vi "Write Excel Files.vi"() -> ()   [LabVIEW 2016]
uses:
  <vilib>/Utility/NIReport.llb/NI_report.lvclass
  sdi_12/Groundwater header.ctl
  <userlib>/_OpenG.lib/file/file.llb/File Exists - Scalar__ogtk.vi
  <userlib>/_OpenG.lib/file/file.llb/Strip Path - Traditional__ogtk.vi
  <vilib>/Utility/file.llb/Write Delimited Spreadsheet (string).vi
  <vilib>/Utility/file.llb/Read Delimited Spreadsheet (string).vi
panel:
  in  "Output path to Directory":path=path "C:/Cascade/Data/Output Files/ara-1"
  in  "Sonde Calibration History File":path
  out "IK Reason array":string[][](array[string])
  in  "Sonde IK Recording Failure Path":path
  out "Recording Reason Sonde array":string[][](array[string])
  in  "Temporary Data Files Directory":path=path "C:/Cascade/Data/Output Files"
  out "KPRO all rows":string[][](array[string])
  out "Sonde Data":string[][](array[string])
  out "Sonde Recording":string[][](array[string])
  out "IK":string[][](array[string])
  out "appended path":path=path "C:/Cascade/Data/Output Files/ara-1/ara-1"
  out "Down hole Pressure Transducer CSV data  path":path=path "C:/Cascade/Data/Output Files/ara-1/ara-1_DHT Data.csv"
  in  "Static IK path":path=path "C:/Cascade/Data/Output Files/ara-1/ara-1_Static Ik.csv"
  out "Output File Path":path=path "C:/Cascade/Data/Output Files/ara-1"
  out "KPRO SessionOutput File Path":path=path "C:/Cascade/Data/Output Files/ara-1/ara-1_KPROsession.csv"
  in  "Sonde Recording Error file":path=path "C:/Cascade/Data/Output Files/ara-1/ara-1_Sample failure.csv"
  in  "IK Recording Error file":path=path "C:/Cascade/Data/Output Files/ara-1/ara-1_IK failure.csv"
  in  "Sonde Output File Path":path=path "C:/Cascade/Data/Output Files/ara-1/ara-1_SondeData.csv"
  in  "KPRO Cumulative Output File Path":path=path "C:/Cascade/Data/Output Files/ara-1/ara-1_KPROcumulative.csv"
  out "error out":errorcluster
  in  "error IO":errorcluster
  in  "Groundwater Header":T1
  in  "Excel report file path":path=path "C:/Cascade/Data/Excel Reports/Groundwater Profiling Log_ara1.xlsx"
  in  "template file path":path=path "C:/Cascade/templates/Groundwater Profiling Log_empty_labview_template.xlsx"
  out "Worksheet Names":string[](array[string])
  out "row max value":i32
  in  "Header path":path=path "C:/Cascade/templates/Fields for Excel sheets.xlsx"
  out "column max value":i32
  out "subarray":string[][](array[string])
  out "NI_report out":refnum<class "NI_report.lvclass">
  out "Number of Sample Sheets":i32
  out "Select Worksheet Index":i32
  out "Columns":i32[](array[numeric])
  out "Column of Volume":i32
  out "last occupied cell's name":string
  in  "Current Sample Sheet":string="Sample 1"
types:
  T1 = typedef "Groundwater header.ctl" = cluster{"Location":string, "Date Finished":string, "CTS":string, "sampler":string, "Kpro box Serial ":string, "Sonde Serial":string, "Drilling Contractor":string, "Ave Depth to Water":string, "Gas/Peri Pump":string, "Atmospheric Pressure":string, "KPRO N2 Pressure":string, "Gas Drive N2 Pressure":string, "Profile ID":string, "Client":string}
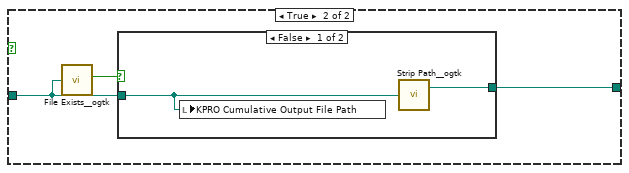
[diagram p2: hidden frame]
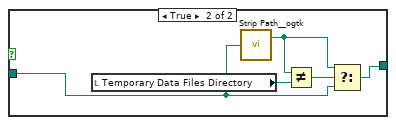
[diagram p3: hidden frame]
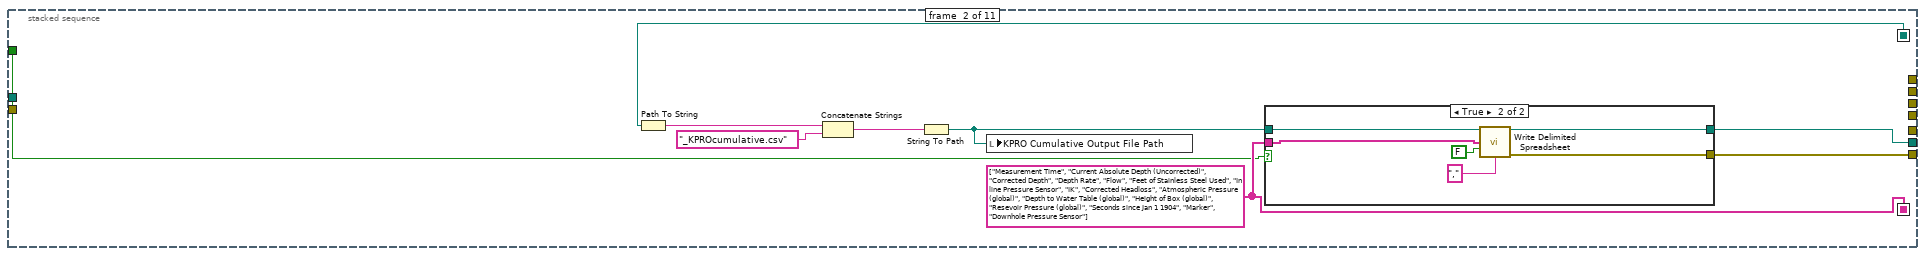
[diagram p4: hidden frame]
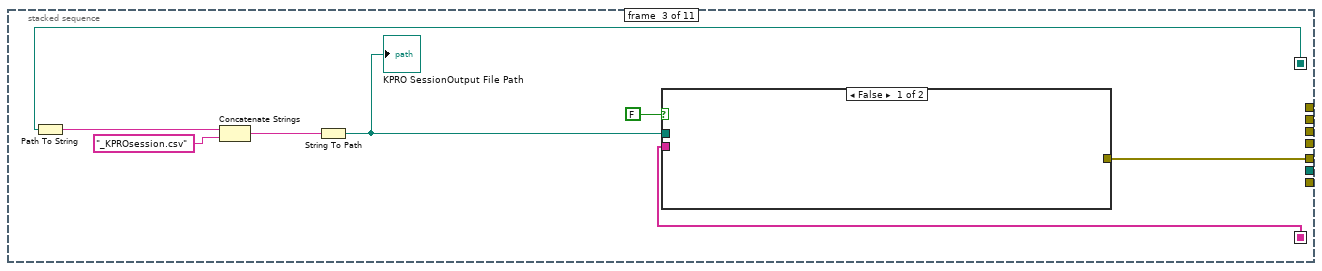
[diagram p6: hidden frame]
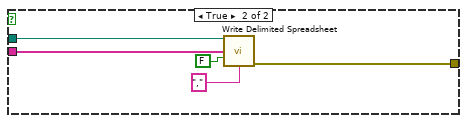
[diagram p7: hidden frame]
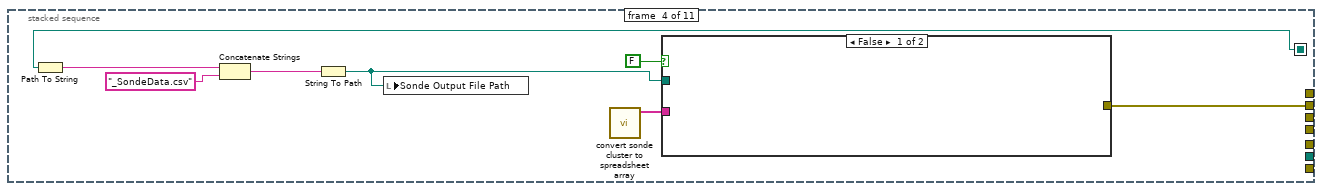
[diagram p8: hidden frame]
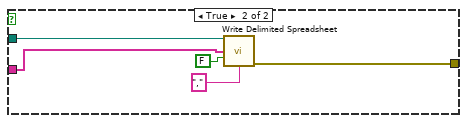
[diagram p9: hidden frame]
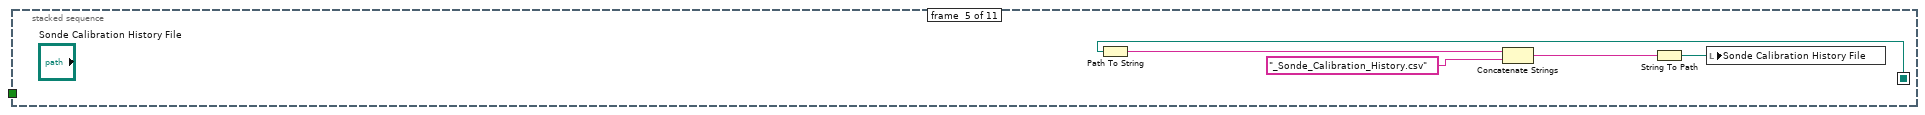
[diagram p10: hidden frame]
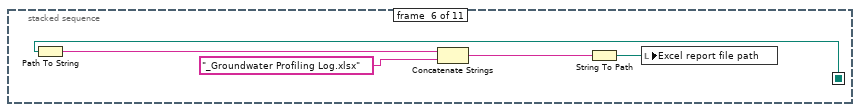
[diagram p11: hidden frame]
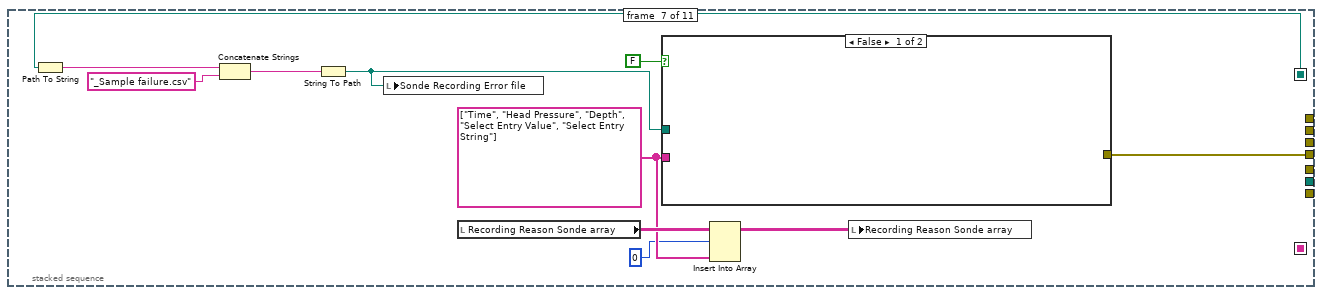
[diagram p12: hidden frame]
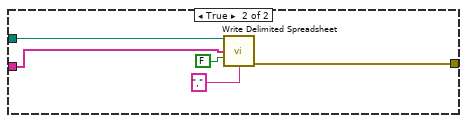
[diagram p13: hidden frame]
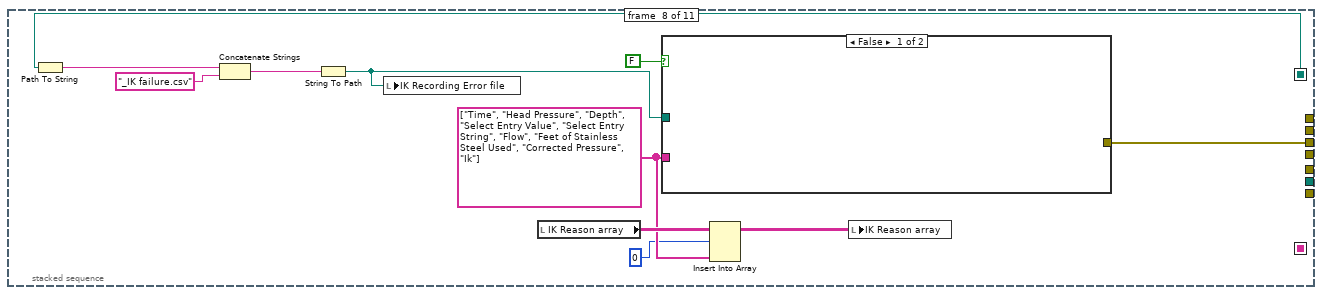
[diagram p14: hidden frame]
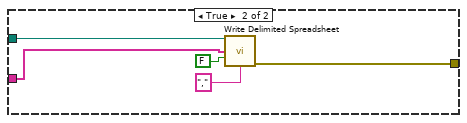
[diagram p15: hidden frame]
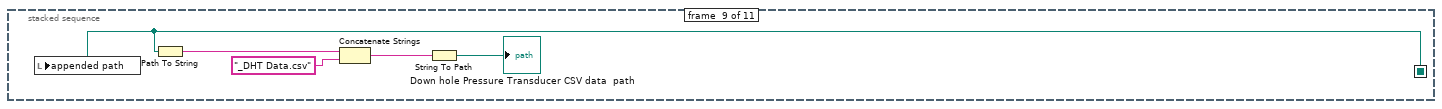
[diagram p16: hidden frame]
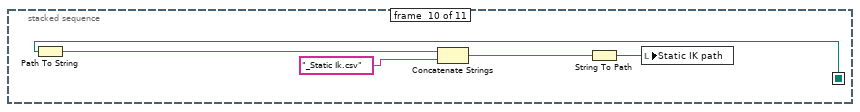
[diagram p17: hidden frame]
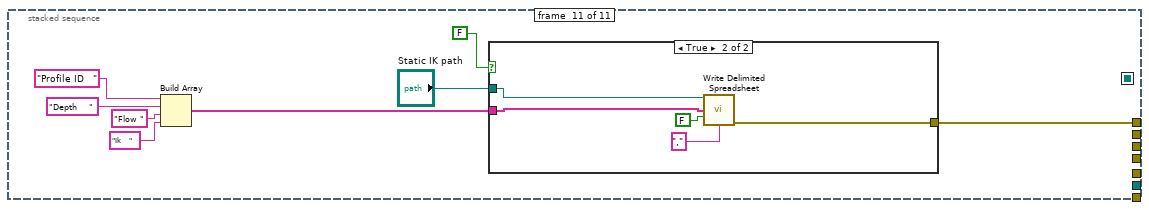
[diagram p18: hidden frame]
diagram:
  w14 = "Groundwater Profile Log" ("Worksheet Name in")
  w31 = "Profile Info" ("Worksheet Name in")
  n1 = stacked-sequence {
    seq-local: [_ w86 _ _ _ _ _ _ _ _ _] -> [_ _ w101 _ _ _ _ _ _ _ _]
    seq-local: [w62 _ _ _ _ _ _ _ _ _ _] -> [_ w87 w102 w114 w125 w130 w141 w157 w168 w172 _]
    tunnel: [_ w84 _ _ _ _ _ _ _ _ _] -> w1
    tunnel: [_ _ w106 _ _ _ _ _ _ _ _] -> _
    tunnel: [_ _ _ w115 _ _ _ _ _ _ _] -> _
    tunnel: [_ _ _ _ _ _ w142 _ _ _ _] -> _
    tunnel: [_ _ _ _ _ _ _ w158 _ _ _] -> _
    tunnel: [_ _ _ _ _ _ _ _ _ _ w179] -> _
    tunnel: [_ w88 _ _ _ _ _ _ _ _ _] -> _
    tunnel: "Output path to Directory" -> [w65 _ _ _ _ _ _ _ _ _ _]
    tunnel: FALSE ("exists") -> [w66 w85 _ _ _ _ _ _ _ _ _]
    tunnel: "error IO" -> [_ _ _ _ _ _ _ _ _ _ _]
    frame #0 {
      n2 = case shown="False" w66 {
        tunnel: w65 -> [w72 w74]
        tunnel: [w72 w73] -> w64
        frame False {
        }
        frame True {
          n3 = call-poly <userlib>:"File Exists__ogtk.vi"("file path"=w74) -> ("is directory"=w75:bool)  [unwired: 6 in, 1 out]
          n4 = case shown="False" w75 {
            tunnel: w74 -> [w76 w78]
            tunnel: [w77 w79] -> w73
            frame False {
              n5 = local write "KPRO Cumulative Output File Path"(w76) -> ()
              n6 = call-poly <userlib>:"Strip Path__ogtk.vi"("path"=w76) -> ("stripped path"=w77:path)  [unwired: 1 out]
            }
            frame True {
              n7 = local read "Temporary Data Files Directory"() -> (w82:path)
              n8 = call-poly <userlib>:"Strip Path__ogtk.vi"("path"=w78) -> ("stripped path"=w80:path)  [unwired: 1 out]
              n9 = Not Equal?(x=w80, y=w82) -> (x != y?=w81:bool)
              n10 = Select(t=w80, s=w81, f=w78) -> (s? t:f=w79:path)
            }
          }
        }
      }
      n11 = Path To String(path=w64) -> (string=w69:string)
      n12 = Concatenate Strings(w69, "\\" ("string")) -> (w70:string)
      n13 = String To Path(string=w70) -> (path=w63:path)
      "Output File Path" <- w63
      n14 = call-poly <userlib>:"Strip Path__ogtk.vi"("path"=w63) -> ("name"=w67:string)  [unwired: 1 out]
      n15 = Concatenate Strings(w70, w67) -> (w68:string)
      n16 = String To Path(string=w68) -> (path=w62:path)
      "appended path" <- w62
    }
    frame #1 {
      w86 = string[] ["Measurement Time", "Current Absolute Depth (Uncorrected)", "Corrected Depth", "Depth Rate", "Flow", "Feet of Stainless Steel Used", "In line Pressure Sensor", "IK", "Corrected Headloss", "Atmospheric Pressure (global)", "Depth to Water Table (global)", "Height of Box (global)", "Resevoir Pressure (global)", "Seconds since Jan 1 1904", "Marker", "Downhole Pressure Sensor"] ("Array")
      n17 = Path To String(path=w87) -> (string=w89:string)
      n18 = Concatenate Strings(w89, "_KPROcumulative.csv") -> (w91:string)
      n19 = String To Path(string=w91) -> (path=w83:path)
      n20 = local write "KPRO Cumulative Output File Path"(w83) -> ()
      n21 = case shown="True" w85 {
        tunnel: [_ w96] -> w84
        tunnel: w83 -> [w92 w95]
        tunnel: [w92 w94] -> w88
        tunnel: w86 -> [_ w93]
        frame False {
        }
        frame True {
          n22 = call-poly <vilib>:"Write Delimited Spreadsheet.vi"("file path (dialog if empty)"=w95, "1D data"=w93, "append to file? (new file:F)"=FALSE, "delimiter (\\t)"="," ("delimiter (\\t)")) -> ("new file path (Not A Path if cancelled)"=w94:path, "error out"=w96:errorcluster)  [unwired: 10 in]
        }
      }
    }
    frame #2 {
      n23 = Path To String(path=w102) -> (string=w104:string)
      n24 = Concatenate Strings(w104, "_KPROsession.csv") -> (w105:string)
      n25 = String To Path(string=w105) -> (path=w100:path)
      "KPRO SessionOutput File Path" <- w100
      n26 = case shown="False" FALSE {
        tunnel: [_ w109] -> w106
        tunnel: w101 -> [_ w108]
        tunnel: w100 -> [_ w107]
        frame False {
        }
        frame True {
          n27 = call-poly <vilib>:"Write Delimited Spreadsheet.vi"("file path (dialog if empty)"=w107, "1D data"=w108, "append to file? (new file:F)"=FALSE, "delimiter (\\t)"="," ("delimiter (\\t)")) -> ("error out"=w109:errorcluster)  [unwired: 10 in, 1 out]
        }
      }
    }
    frame #3 {
      n28 = Path To String(path=w114) -> (string=w117:string)
      n29 = Concatenate Strings(w117, "_SondeData.csv" ("string")) -> (w118:string)
      n30 = String To Path(string=w118) -> (path=w113:path)
      n31 = local write "Sonde Output File Path"(w113) -> ()
      n32 = call "convert sonde cluster to spreadsheet array.vi"() -> ("sonde labels"=w116:string[])  [unwired: 8 in, 3 out]
      n33 = case shown="False" FALSE {
        tunnel: w116 -> [_ w124]
        tunnel: [_ w121] -> w115
        tunnel: w113 -> [_ w120]
        frame False {
        }
        frame True {
          n34 = call-poly <vilib>:"Write Delimited Spreadsheet.vi"("file path (dialog if empty)"=w120, "1D data"=w124, "append to file? (new file:F)"=FALSE, "delimiter (\\t)"="," ("delimiter (\\t)")) -> ("error out"=w121:errorcluster)  [unwired: 10 in, 1 out]
        }
      }
    }
    frame #4 {
      n35 = Path To String(path=w125) -> (string=w127:string)
      n36 = Concatenate Strings(w127, "_Sonde_Calibration_History.csv" ("string")) -> (w128:string)
      n37 = String To Path(string=w128) -> (path=w126:path)
      n38 = local write "Sonde Calibration History File"(w126) -> ()
    }
    frame #5 {
      n39 = Path To String(path=w130) -> (string=w132:string)
      n40 = Concatenate Strings(w132, "_Groundwater Profiling Log.xlsx" ("string")) -> (w133:string)
      n41 = String To Path(string=w133) -> (path=w131:path)
      n42 = local write "Excel report file path"(w131) -> ()
    }
    frame #6 {
      w138 = string[] ["Time", "Head Pressure", "Depth", "Select Entry Value", "Select Entry String"]
      n43 = Path To String(path=w141) -> (string=w143:string)
      n44 = Concatenate Strings(w143, "_Sample failure.csv" ("new ending (none)")) -> (w144:string)
      n45 = String To Path(string=w144) -> (path=w136:path)
      n46 = local write "Sonde Recording Error file"(w136) -> ()
      n47 = local read "Recording Reason Sonde array"() -> (w139:string[][])
      n48 = case shown="False" FALSE {
        tunnel: [_ w148] -> w142
        tunnel: w138 -> [_ w147]
        tunnel: w136 -> [_ w146]
        frame False {
        }
        frame True {
          n49 = call-poly <vilib>:"Write Delimited Spreadsheet.vi"("file path (dialog if empty)"=w146, "1D data"=w147, "append to file? (new file:F)"=FALSE, "delimiter (\\t)"="," ("delimiter (\\t)")) -> ("error out"=w148:errorcluster)  [unwired: 10 in, 1 out]
        }
      }
      n50 = Insert Into Array(array=w139, index (row)=0, new element=w138) -> (w140:string[][])  [unwired: 1 in]
      n51 = local write "Recording Reason Sonde array"(w140) -> ()
    }
    frame #7 {
      w154 = string[] ["Time", "Head Pressure", "Depth", "Select Entry Value", "Select Entry String", "Flow", "Feet of Stainless Steel Used", "Corrected Pressure", "Ik"]
      n52 = Path To String(path=w157) -> (string=w159:string)
      n53 = Concatenate Strings(w159, "_IK failure.csv" ("new ending (none)")) -> (w160:string)
      n54 = String To Path(string=w160) -> (path=w152:path)
      n55 = local write "IK Recording Error file"(w152) -> ()
      n56 = local read "IK Reason array"() -> (w155:string[][])
      n57 = case shown="False" FALSE {
        tunnel: [_ w164] -> w158
        tunnel: w154 -> [_ w163]
        tunnel: w152 -> [_ w162]
        frame False {
        }
        frame True {
          n58 = call-poly <vilib>:"Write Delimited Spreadsheet.vi"("file path (dialog if empty)"=w162, "1D data"=w163, "append to file? (new file:F)"=FALSE, "delimiter (\\t)"="," ("delimiter (\\t)")) -> ("error out"=w164:errorcluster)  [unwired: 10 in, 1 out]
        }
      }
      n59 = Insert Into Array(array=w155, index (row)=0, new element=w154) -> (w156:string[][])  [unwired: 1 in]
      n60 = local write "IK Reason array"(w156) -> ()
    }
    frame #8 {
      n61 = local write "appended path"(w168) -> ()
      n62 = Path To String(path=w168) -> (string=w169:string)
      n63 = Concatenate Strings(w169, "_DHT Data.csv" ("new ending (none)")) -> (w170:string)
      n64 = String To Path(string=w170) -> (path=→"Down hole Pressure Transducer CSV data  path":path)
    }
    frame #9 {
      n65 = Path To String(path=w172) -> (string=w173:string)
      n66 = Concatenate Strings(w173, "_Static Ik.csv" ("string")) -> (w175:string)
      n67 = String To Path(string=w175) -> (path=w174:path)
      n68 = local write "Static IK path"(w174) -> ()
    }
    frame #10 {
      n69 = Build Array("Profile ID   " ("string"), "Depth    " ("string"), "Flow " ("string"), "Ik    " ("string")) -> (w180:string[])
      n70 = case shown="True" FALSE {
        tunnel: w180 -> [_ w188]
        tunnel: [_ w186] -> w179
        tunnel: "Static IK path" -> [_ w185]
        frame False {
        }
        frame True {
          n71 = call-poly <vilib>:"Write Delimited Spreadsheet.vi"("file path (dialog if empty)"=w185, "1D data"=w188, "append to file? (new file:F)"=FALSE, "delimiter (\\t)"="," ("delimiter (\\t)")) -> ("error out"=w186:errorcluster)  [unwired: 10 in, 1 out]
        }
      }
    }
  }
  n72 = flat-sequence {
    tunnel: [w205] -> w40
    tunnel: [w204] -> _
    tunnel: [w194] -> _
    tunnel: [w202] -> _
    tunnel: [w201] -> w61
    tunnel: [w200] -> w60
    tunnel: [w198] -> _
    tunnel: w1 -> [w192]
    frame #0 {
      n73 = call "setup excel worksheet.vi"("Current Sample Sheet"="Current Sample Sheet", "template file path"="template file path", "Excel report file path"="Excel report file path", "error in (no error)"=w192, "Header path"="Header path", "Open Excel Files"=TRUE) -> ("subarray"=→"subarray":string[][], "column max value"=→"column max value":i32, "row max value"=→"row max value":i32, "Column of Volume"=w198:i32, "Worksheet Names"=w194:string[], "NI_report out"=w201:refnum<class "NI_report.lvclass">, "Columns"=w204:i32[], "start of last occupied row"=→"last occupied cell's name":string, "Number of Sample Sheets"=w205:i32, "Select Worksheet Index"=w202:i32, "error out"=w200:errorcluster)  [unwired: 3 in]
      "Worksheet Names" <- w194
      "NI_report out" <- w201
      "Number of Sample Sheets" <- w205
      "Select Worksheet Index" <- w202
      "Columns" <- w204
      "Column of Volume" <- w198
    }
  }
  n74 = call <vilib>:"Clear Errors.vi"("error in (no error)"=w60) -> ("error out"=w5:errorcluster)  [unwired: 5 in, 1 out]
  n75 = local read "Worksheet Names"() -> (w12:string[])
  n76 = Get Date/Time In Seconds() -> (seconds since 1Jan1904=w9:timestamp)
  n77 = Get Date/Time String(seconds (now)=w9) -> (date string=w7:string)  [unwired: 2 in, 1 out]
  n78 = local write "Current Sample Sheet"(w14) -> ()
  n79 = Bundle By Name(cluster="Groundwater Header", "Date Finished"=w7) -> (w8:T1)
  n80 = call "find and open select worksheet.vi"("Worksheet Names"=w12, "error in (no error)"=w5, "milliseconds to wait"=u32 100, "Worksheet Name in"=w14, "NI_report in"=w61) -> ("error out"=w11:errorcluster, "NI_report out"=w10:refnum<class "NI_report.lvclass">)  [unwired: 4 in, 1 out]
  n81 = call "groundwater log header.vi"("Worksheet Names"=w12, "Groundwater Header"=w8, "error in (no error)"=w11, "NI_report in"=w10) -> ("error out"=w56:errorcluster, "NI_report out"=w57:refnum<class "NI_report.lvclass">)  [unwired: 6 in]
  n82 = local read "Worksheet Names"() -> (w29:string[])
  n83 = local write "Current Sample Sheet"(w31) -> ()
  n84 = call "find and open select worksheet.vi"("Worksheet Names"=w29, "error in (no error)"=w56, "milliseconds to wait"=u32 100, "Worksheet Name in"=w31, "NI_report in"=w57) -> ("error out"=w24:errorcluster, "NI_report out"=w25:refnum<class "NI_report.lvclass">)  [unwired: 4 in, 1 out]
  n85 = call "Read Recording Error File Write Cells.vi"("Reason Column Letter"="D", "Depth Column Letter"="C", "error in (no error)"=w24, "Row Offset In"=16, "Sonde Data file"="IK Recording Error file", "NI_report in"=w25) -> ("error out"=w22:errorcluster, "all rows"=→"IK":string[][], "Row Offset Out"=w20:i32, "NI_report out"=w23:refnum<class "NI_report.lvclass">)  [unwired: 2 in]
  n86 = call "Read Recording Error File Write Cells.vi"("Reason Column Letter"="F", "error in (no error)"=w22, "Row Offset In"=w20, "Sonde Data file"="Sonde Recording Error file", "NI_report in"=w23) -> ("error out"=w49:errorcluster, "all rows"=→"Sonde Recording":string[][], "NI_report out"=w51:refnum<class "NI_report.lvclass">)  [unwired: 3 in, 1 out]
  n87 = call <vilib>:"Clear Errors.vi"("error in (no error)"=w49) -> ("error out"=w46:errorcluster)  [unwired: 5 in, 1 out]
  n88 = call "get sonde data.vi"("error in (no error)"=w46, "Sonde Output File Path"="Sonde Output File Path") -> ("error out"=w48:errorcluster, "Sample Row \nBreak points"=w47:i32[], "Sample Array"=w39:i32[], "Sonde Data"=w50:string[][])  [unwired: 6 in]
  "Sonde Data" <- w50
  n89 = local read "Worksheet Names"() -> (w41:string[])
  n90 = call "Write Sonde Data cells to excel.vi"("NI_report in"=w51, "all rows"=w50, "error in (no error)"=w48, "Worksheet Names"=w41, "Sample Array"=w39, "Sample Row \nBreak points"=w47, "Number of Sample Sheets"=w40) -> ("NI_report out"=w35:refnum<class "NI_report.lvclass">, "error out"=w44:errorcluster)  [unwired: 10 in, 1 out]
  n91 = call <vilib>:"Clear Errors.vi"("error in (no error)"=w44) -> ("error out"=w37:errorcluster)  [unwired: 5 in, 1 out]
  n92 = call-poly <vilib>:"Read Delimited Spreadsheet.vi"("file path (dialog if empty)"="KPRO Cumulative Output File Path", "error in (no error)"=w37, "delimiter (\\t)"="," ("delimiter (\\t)")) -> ("all rows"=w42:string[][], "error out"=w43:errorcluster)  [unwired: 7 in, 4 out]
  "KPRO all rows" <- w42
  n93 = call "Write KPRO Data cells to excel.vi"("NI_report in"=w35, "all rows"=w42, "Row Offset In"=2, "error in (no error)"=w43, "Worksheet Names"=w41) -> ("NI_report out"=w34:refnum<class "NI_report.lvclass">, "error out"=w38:errorcluster)  [unwired: 12 in, 1 out]
  n94 = call <vilib>:"Clear Errors.vi"("error in (no error)"=w38) -> ("error out"=w36:errorcluster)  [unwired: 5 in, 1 out]
  n95 = flat-sequence {
    tunnel: w36 -> [w216]
    tunnel: [w215] -> w59
    tunnel: w34 -> [w214]
    tunnel: [w213] -> w58
    tunnel: w40 -> [w209]
    tunnel: w41 -> [w207]
    frame #0 {
      # "Disabled"
      n96 = call "open select sample sheet.vi"("Number of Sample Sheets"=w209, "error in (no error)"=w216, "Worksheet Names"=w207, "input 1"=0 ("Active Sample Sheet"), "NI_report in"=w214) -> ("error out"=w212:errorcluster, "Current Sample Sheet"=w208:string, "NI_report out"=w211:refnum<class "NI_report.lvclass">)  [unwired: 4 in]
      n97 = flat-sequence {
        tunnel: [w228] -> w213
        tunnel: [w227] -> _
        tunnel: w212 -> [w226]
        tunnel: [w219] -> w215
        tunnel: w208 -> [w218]
        tunnel: w211 -> [w217]
        frame #0 {
          n98 = call "get sample sheet data cells.vi"("error in (no error)"=w226, "NI_report in"=w217) -> ("error out"=w229:errorcluster, "data"=w224:string[][], "NI_report out"=w228:refnum<class "NI_report.lvclass">, "left edge output cluster"=w222:cluster{"row":i32, "column":i32})  [unwired: 5 in, 1 out]
          n99 = call "find last occupied cell.vi"("Active Sheet"=w218, "Header Rows to remove"=3, "sub array start"=w222, "error in (no error)"=w229) -> ("row max value"=w221:i32, 13:"start of last occupied row"=w227:cluster{"row":i32, "column":i32}, 14:"start of last occupied row"=w220:string, "error out"=w219:errorcluster)  [unwired: 5 in, 3 out]
          n100 = Array Subset(array=w224, index (col)=2 ("index")) -> ()  [unwired: 3 in, 1 out]
          n101 = local write "row max value"(w221) -> ()
          n102 = local write "last occupied cell's name"(w220) -> ()
        }
      }
      n103 = local write "Current Sample Sheet"(w208) -> ()
    }
  }
  n104 = call <vilib>:"Clear Errors.vi"("error in (no error)"=w59) -> ("error out"=w6:errorcluster)  [unwired: 5 in, 1 out]
  n105 = flat-sequence {
    tunnel: [w235] -> w55
    tunnel: [w234] -> w54
    tunnel: w6 -> [w232]
    tunnel: w58 -> [w231]
    frame #0 {
      n106 = local read "Excel report file path"() -> (w230:path)
      n107 = call-dynamic "Save Report to File.vi"("report in"=w231, "report file path"=w230, "prompt to replace? (F)"=FALSE, "error in (no error)"=w232) -> ("report out"=w235:refnum<class "NI_report.lvclass">, "error out"=w234:errorcluster)  [unwired: 10 in]
    }
  }
  n108 = call-dynamic "Dispose Report.vi"("report in"=w55, "error in (no error)"=w54) -> ("error out"=→"error out":errorcluster)  [unwired: 13 in]
